vi "clawControl.vi"(9 "open":bool, 11 "up":bool) -> ()   [LabVIEW 2017]
uses:
  <vilib>/Rock Robotics/WPI/Solenoid/WPI_SolenoidValue.ctl
  <vilib>/Rock Robotics/Network Tables/NT Write Boolean.vi
  <vilib>/Rock Robotics/WPI/Solenoid/WPI_SolenoidSetEnum.vi
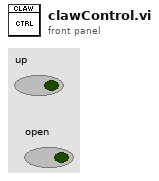
[diagram p1: front panel]
types:
  T1 = typedef "WPI_SolenoidValue.ctl" = enum16{"Off", "On", "Forward", "Reverse"}
  T2 = typedef "WPI_SolenoidDevRef.ctl" = cluster{"DevStatus":errorcluster, "Pneumatics Control Module":u8, "Forward Solenoid Channel":T3, "Reverse Solenoid Channel":T3}
  T3 = typedef "WPI_SolenoidChannel.ctl" = enum8{"Solenoid 0", "Solenoid 1", "Solenoid 2", "Solenoid 3", "Solenoid 4", "Solenoid 5", "Solenoid 6", "Solenoid 7", "Invalid"}
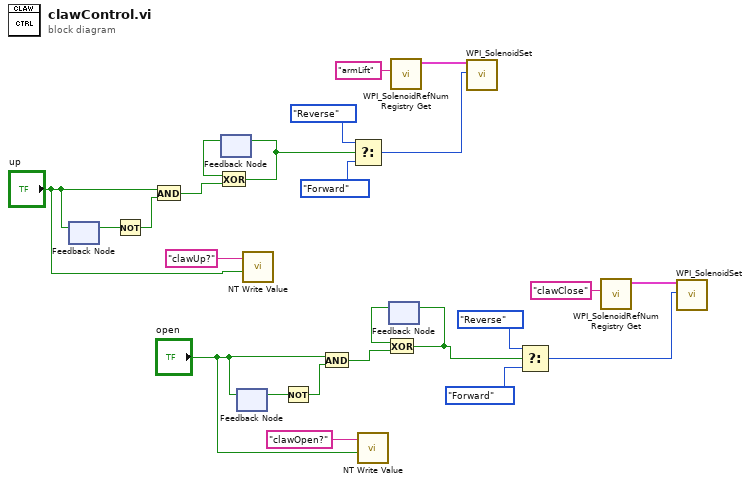
[diagram p0: block diagram]
diagram:
  n1 = feedback #1() -> (w8:bool)  [unwired: 1 in]
  n2 = feedback-in #1("up") -> ()
  n3 = Not(x=w8) -> (.not. x?=w7:bool)
  n4 = And(x="up", y=w7) -> (x .and. y?=w6:bool)
  n5 = feedback #2() -> (w9:bool)  [unwired: 1 in]
  n6 = Exclusive Or(1:w6, 2:w9) -> (0:w5:bool)
  n7 = feedback-in #2(w5) -> ()
  n8 = feedback-in #3("open") -> ()
  n9 = feedback #3() -> (w14:bool)  [unwired: 1 in]
  n10 = call-poly <vilib>:"NT Write Value.vi"("Boolean"="up", "Name"="clawUp?") -> ()  [unwired: 9 in, 1 out]
  n11 = Not(x=w14) -> (.not. x?=w15:bool)
  n12 = And(x="open", y=w15) -> (x .and. y?=w16:bool)
  n13 = Select(t=WPI_SolenoidValue."Reverse", s=w5, f=WPI_SolenoidValue."Forward") -> (s? t:f=w10:T1)
  n14 = call-poly <vilib>:"NT Write Value.vi"("Boolean"="open", "Name"="clawOpen?") -> ()  [unwired: 9 in, 1 out]
  n15 = feedback #4() -> (w12:bool)  [unwired: 1 in]
  n16 = Exclusive Or(1:w16, 2:w12) -> (0:w13:bool)
  n17 = feedback-in #4(w13) -> ()
  n18 = call <vilib>:"WPI_SolenoidRefNum Registry Get.vi"("refnum name"="armLift") -> ("SolenoidDevRef"=w23:T2)  [unwired: 9 in, 1 out]
  n19 = call-poly <vilib>:"WPI_SolenoidSet.vi"("Value"=w10, "SolenoidDevRef"=w23) -> ()  [unwired: 8 in, 2 out]
  n20 = Select(t=WPI_SolenoidValue."Reverse", s=w13, f=WPI_SolenoidValue."Forward") -> (s? t:f=w19:T1)
  n21 = call <vilib>:"WPI_SolenoidRefNum Registry Get.vi"("refnum name"="clawClose") -> ("SolenoidDevRef"=w20:T2)  [unwired: 9 in, 1 out]
  n22 = call-poly <vilib>:"WPI_SolenoidSet.vi"("Value"=w19, "SolenoidDevRef"=w20) -> ()  [unwired: 8 in, 2 out]
